vi "Quick Usb Get Driver Version.vi"(8 "error in (no error)":errorcluster, 9 "BuildDriverVersion":u16, 10 "MinorDriverVersion":u16, 11 "MajorDriverVersion":u16) -> (0 "error out":errorcluster, 1 "BuildDriverVersion out":u16, 2 "MinorDriverVersion out":u16, 3 "MajorDriverVersion out":u16, 5 "function return":i32)   [LabVIEW 2011, in "QuickUSB.lvlib"]
doc: "QUSBLIB QRETURN QuickUsbGetDriverVersion(\n PQWORD MajorDriverVersion,\n PQWORD MinorDriverVersion,\n PQWORD BuildDriverVersion\n);"
uses:
  QuickUSB.lvlib
  QuickUSB.dll
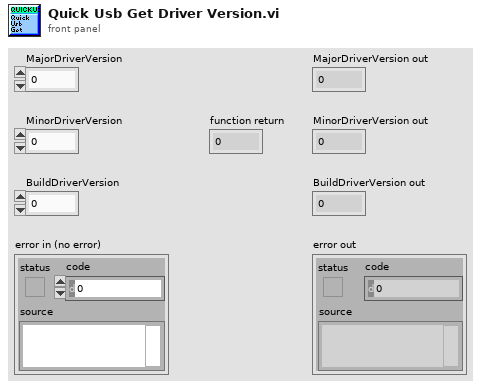
[diagram p1: front panel]
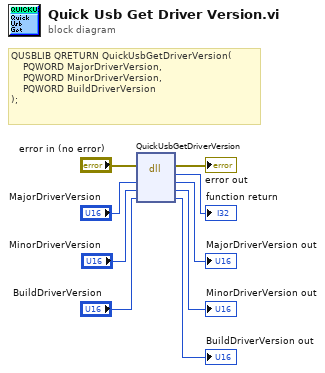
[diagram p0: block diagram]
diagram:
  # "QUSBLIB QRETURN QuickUsbGetDriverVersion(\n    PQWORD MajorDriverVersion,\n    PQWORD MinorDriverVersion,\n    PQWORD BuildDriverVersion\n);"
  n1 = dll-call lib="C:/QuickUSB/QuickUSB.*" fn="QuickUsbGetDriverVersion"(error in="error in (no error)", "MajorDriverVersion"="MajorDriverVersion", "MinorDriverVersion"="MinorDriverVersion", "BuildDriverVersion"="BuildDriverVersion") -> (error out=→"error out":errorcluster, →"function return":i32, "MajorDriverVersion"=→"MajorDriverVersion out":u16, "MinorDriverVersion"=→"MinorDriverVersion out":u16, "BuildDriverVersion"=→"BuildDriverVersion out":u16)  [unwired: 2 in, 1 out]
